vi "Simulação Controlo PID.vi"() -> ()   [LabVIEW 2021]
uses:
  <vilib>/addons/control/pid/pid.llb/PID (DBL).vi
  <vilib>/addons/control/pid/NI_PID_pid.lvlib
panel:
  in  "PID gains":T1={"proportional gain (Kc)"=1.0, "integral time (Ti, min)"=0.01, "derivative time (Td, min)"=0.0} {"derivative time (Td, min)" format="%.3f"; "integral time (Ti, min)" format="%.3f"; "proportional gain (Kc)" format="%.3f"}
  in  "Disturbance":dbl(slide)=10.0 min=10.0 max=20.0 step=0.10000000149011612 scale=10.0..20.0 scale format="%.1f"
  in  "Set Point":dbl(slide) scale=0.0..100.0
  out "?":cluster{"Set Point":dbl, "Process Value":dbl}(graph)
  in  "stop":bool
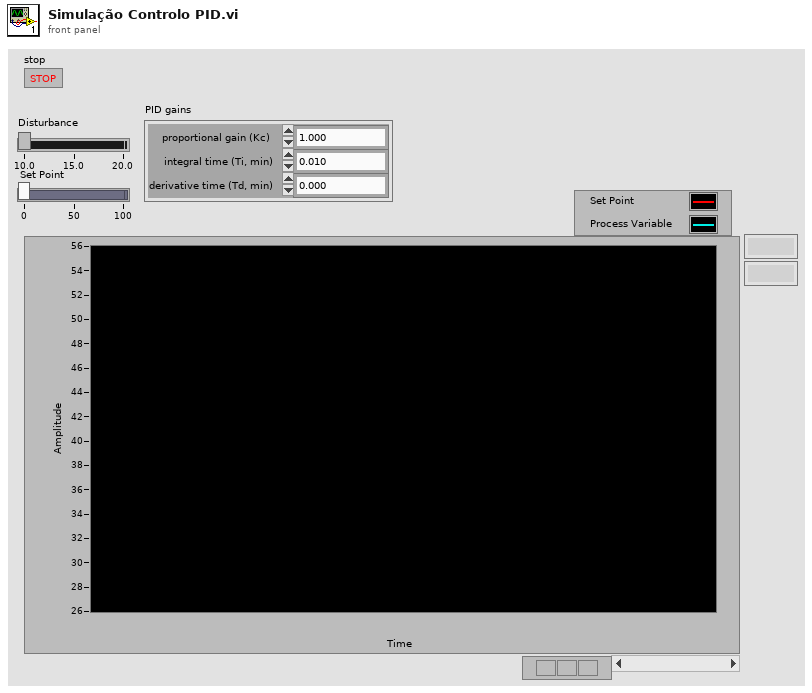
[diagram p1: front panel]
types:
  T1 = cluster{"proportional gain (Kc)":dbl, "integral time (Ti, min)":dbl, "derivative time (Td, min)":dbl}
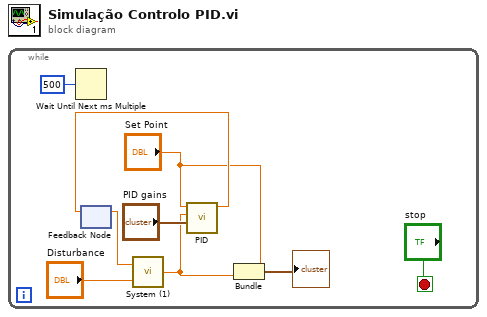
[diagram p0: block diagram]
diagram:
  n1 = while {
    stop <- "stop" stop-if-true
    n2 = Wait Until Next ms Multiple(millisecond multiple=u32 500 ("milliseconds to wait")) -> ()  [unwired: 1 out]
    n3 = feedback #1() -> (w6:dbl)  [unwired: 1 in]
    n4 = call "System (1).vi"("Disturbance"="Disturbance", "Control Action"=w6) -> ("Process Value"=w3:dbl)
    n5 = call-poly <vilib>:"PID.vi"("PID gains"="PID gains", "process variable"=w3, "setpoint"="Set Point") -> ("output"=w7:dbl)  [unwired: 7 in, 1 out]
    n6 = feedback-in #1(w7) -> ()
    n7 = Bundle("Set Point"="Set Point", "Process Value"=w3) -> (→"?":cluster{"Set Point":dbl, "Process Value":dbl})  [unwired: 1 in]
  }
